vi "test_sum_ASIC.vi"() -> ()   [LabVIEW 2009]
uses:
  <vilib>/Utility/NIReport.llb/NI_report.lvclass
  <vilib>/Utility/NIReport.llb/HTML/NI_HTML.lvclass
panel:
  in  "IB_Clip":i32[](array[numeric])=[63, 61, 59, 57, 55, 53, 51, 49, 47, 45, 43, 41, 39, 37, 35, 33, 31, 29, 27, 25, 23, 21, 19, 17, 15, 13, 11, 9, 7, 5, 3, 1]
  in  "Voltages comprobation test":dbl[](array[numeric])=[0.05, 0.2, 0.4, 0.6, 1.0]
  in  "Adds":bool=TRUE
  in  "Full test":bool=TRUE
  out "error out":errorcluster
  out "Instrument VISA out":T1={"AWG VISA"="generadorpulsos", "Oscilloscope  VISA "="Oscilloscope", "Integration Board IP"="172.16.7.43", "connection ID"=refnum, "report out"=refnum, "report file path"=path "D:/CTA/Data_test/ASIC/test3a"}
  in  "Save NOW!":bool
  in  "Instrument VISA in":T1={"AWG VISA"="generadorpulsos", "Oscilloscope  VISA "="Oscilloscope", "Integration Board IP"="172.16.7.43", "connection ID"=refnum, "report out"=refnum, "report file path"=path "D:/CTA/Data_test/ASIC/chip19"}
  in  "error in":errorcluster
  in  "Att_gain_b":i32[](array[numeric])=[0, 1, 2, 3, 4, 5, 6, 7, 8, 9, 10, 11, 12, 13, 14, 15]
  in  "Clip_sel":i32[](array[numeric])=[1, 2, 3]
  in  "Channels":i32[](array[numeric])=[0, 1, 2, 3, 4, 5, 6]
  in  "Voltages comprobation":dbl[](array[numeric])=[0.05, 0.1, 0.2, 0.3, 0.4, 0.5, 0.6, 0.7, 0.8, 1.0]
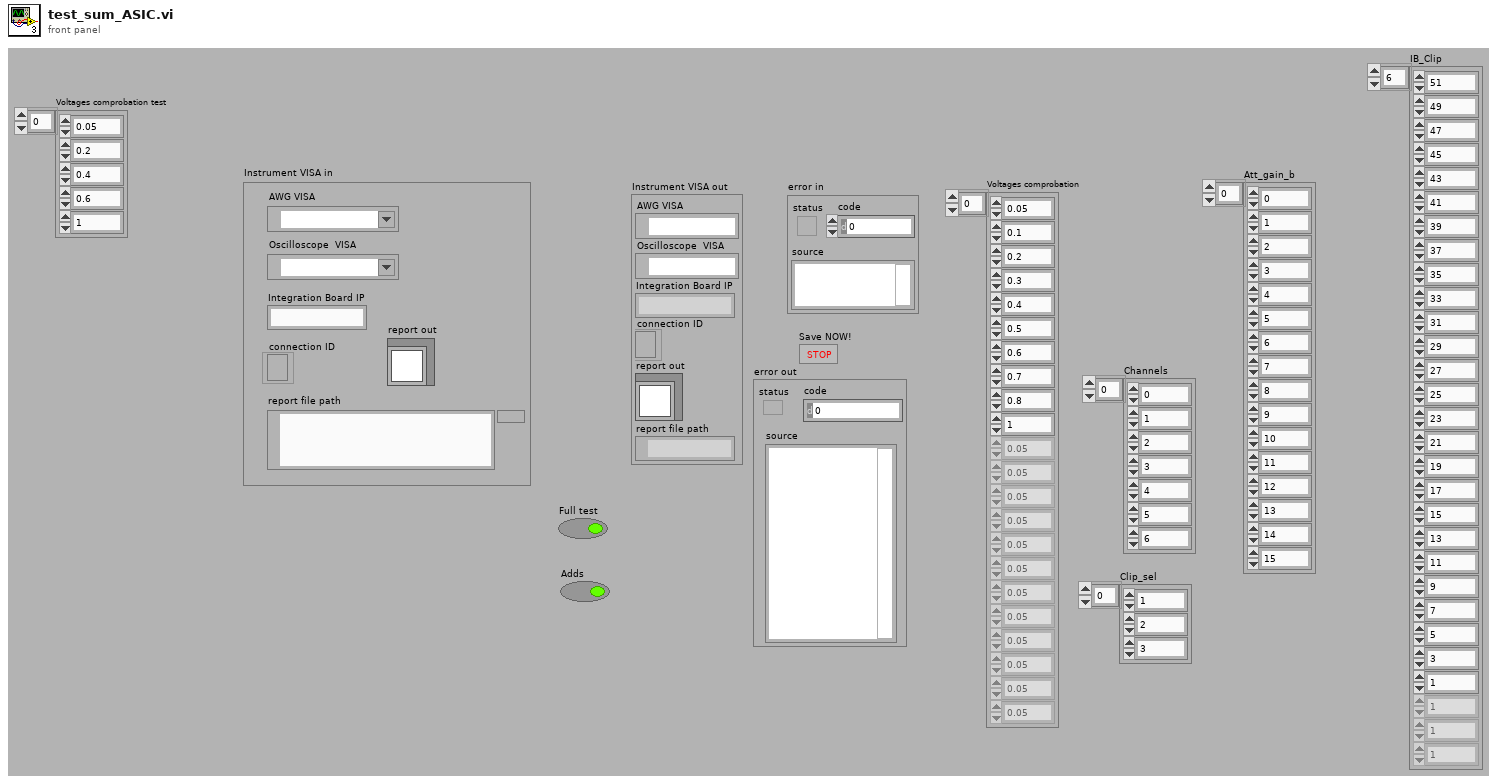
[diagram p1: front panel]
types:
  T1 = cluster{"AWG VISA":refnum<visa-resource-name>, "Oscilloscope  VISA ":refnum<visa-resource-name>, "Integration Board IP":string, "connection ID":refnum<k5>, "report out":refnum<class "NI_report.lvclass">, "report file path":path}
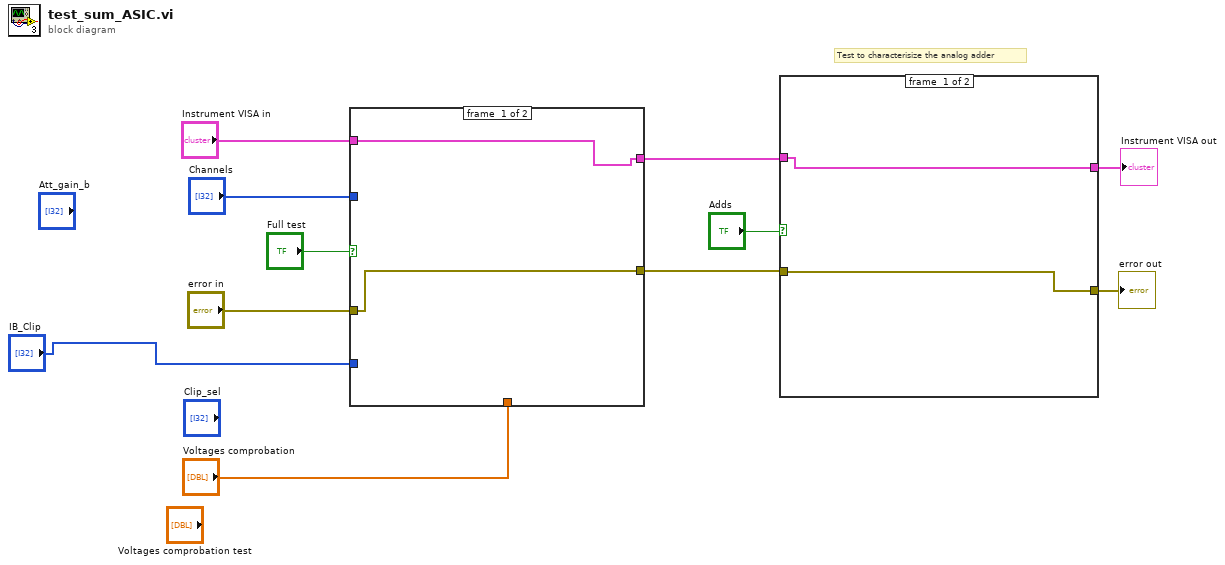
[diagram p0: block diagram]
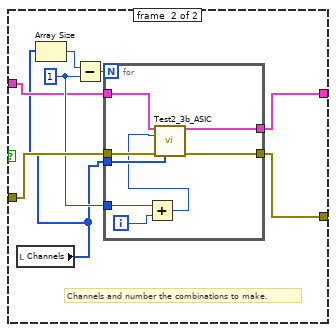
[diagram p2: hidden frame]
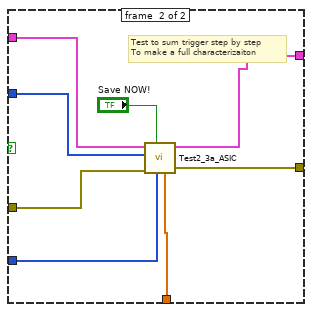
[diagram p3: hidden frame]
diagram:
  # "Test to characterisize the analog adder"
  n1 = case shown="True" "Full test" {
    tunnel: "Voltages comprobation" -> [_ w21]
    tunnel: "error in" -> [w13 w20]
    tunnel: "Channels" -> [_ w19]
    tunnel: "Instrument VISA in" -> [w12 w18]
    tunnel: "IB_Clip" -> [_ w17]
    tunnel: [w13 w15] -> w9
    tunnel: [w12 w14] -> w6
    frame #0 {
    }
    frame #1 {
      # "Test to sum trigger step by step\nTo make a full characterizaiton"
      n2 = call "Test2_3a_ASIC.vi"("Voltages comprobation"=w21, "IB_Clip"=w17, "Save NOW!"="Save NOW!", "error in"=w20, "Channels"=w19, "Instrument VISA in"=w18) -> ("error out"=w15:errorcluster, "Instrument VISA out"=w14:T1)  [unwired: 4 in]
    }
  }
  n3 = case shown="True" "Adds" {
    tunnel: [w22 w31] -> w7
    tunnel: [w23 w29] -> w8
    tunnel: w9 -> [w23 w30]
    tunnel: w6 -> [w22 w25]
    frame #0 {
    }
    frame #1 {
      w26 = 1 ("y")
      # "Channels and number the combinations to make."
      n4 = local read "Channels"() -> (w24:i32[])
      n5 = Array Size(array=w24) -> (size(s)=w27:i32)
      n6 = Subtract(x=w27, y=w26) -> (x-y=w28:i32)
      n7 = for {
        N: w28 -> [_]
        tunnel: [w39] -> w31
        tunnel: w25 -> [w38]
        tunnel: w30 -> [w37]
        tunnel: [w36] -> w29
        tunnel: w24 -> [w35]
        tunnel: w26 -> [w33]
        i -> [w34]
        n8 = Add(x=w33, y=w34) -> (x+y=w32:i32)
        n9 = call "Test2_3b_ASIC.vi"("Instrument VISA in"=w38, "quantity"=w32, "error in"=w37, "channel array"=w35) -> ("Instrument VISA out"=w39:T1, "error out"=w36:errorcluster)  [unwired: 10 in]
      }
    }
  }
  "Instrument VISA out" <- w7
  "error out" <- w8
